vi "Temperature Event Example.vi"() -> ()   [LabVIEW 2012, in "Phidget Temperature Sensor.lvlib"]
uses:
  <instrlib>/Phidgets/Phidget Temperature Sensor/Phidget Temperature Sensor.lvlib
  <instrlib>/Phidgets/Phidget Temperature Sensor/Public/TemperatureSensorStart.vi
  <instrlib>/Phidgets/Phidget Temperature Sensor/Public/TemperatureSensorClose.vi
  <instrlib>/Phidgets/Phidget Common/Phidget Common.lvlib
panel:
  out "Temperature":dbl
  in  "stop":bool
  out "Serial Number Return":i32
  in  "Device Info":T1={"Serial Number"=-1, "Channel"=0, "Port"=0}
  out "error out":errorcluster
  # "Be sure to use this stop button to stop the program.\nIf you use the \"Abort Execution\" button, you will\nneed to use PhidgetResetLibrary.vi or restart Labview \nin order for any Phidgets to work."
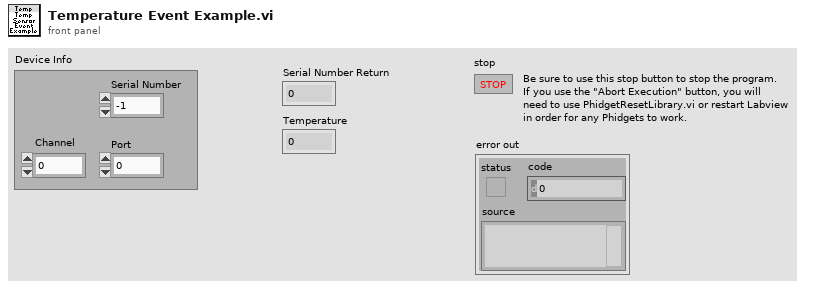
[diagram p1: front panel]
types:
  T1 = cluster{"Serial Number":i32, "Channel":i32, "Port":i32}
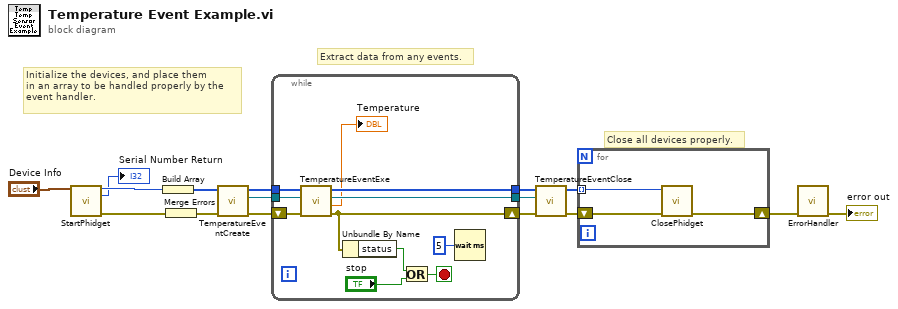
[diagram p0: block diagram]
diagram:
  # "Close all devices properly."
  # "Extract data from any events."
  # "Initialize the devices, and place them\nin an array to be handled properly by the\nevent handler."
  n1 = call-poly <instrlib>:"StartPhidget.vi"("Device Info"="Device Info") -> ("Phidget ID"=w6:u64, "Serial Number Return"=→"Serial Number Return":i32, "error out"=w2:errorcluster)  [unwired: 11 in, 1 out]
  n2 = Build Array(w6) -> (w16:u64[])
  n3 = Merge Errors(w2) -> (w8:errorcluster)
  n4 = call <instrlib>:"TemperatureEventCreate.vi"("error in (no error)"=w8, "Devices In"=w16) -> ("error out"=w10:errorcluster, "Event Registration Refnum"=w3:refnum<event-registration>, "Devices Out"=w15:u64[])  [unwired: 7 in]
  n5 = while {
    tunnel: w15 -> [w27]
    tunnel: [w26] -> w12
    shift-right: [w22] -> w11
    shift-left: w10 -> [w25]
    tunnel: [w23] -> w4
    tunnel: w3 -> [w18]
    stop <- w21 stop-if-true
    n6 = call <instrlib>:"TemperatureEventExe.vi"("error in (no error)"=w25, "Event Registration Refnum In"=w18, "Devices In"=w27) -> ("error out"=w22:errorcluster, "Temperature"=→"Temperature":dbl, "Event Registration Refnum Out"=w26:refnum<event-registration>, "Devices Out"=w23:u64[])  [unwired: 3 in, 2 out]
    n7 = Unbundle By Name(w22) -> ("status"=w19:bool)
    n8 = Or(x=w19, y="stop") -> (x .or. y?=w21:bool)
    n9 = Wait (ms)(milliseconds to wait=u32 5) -> ()  [unwired: 1 out]
  }
  n10 = call <instrlib>:"TemperatureEventClose.vi"("error in (no error)"=w11, "Event Registration Refnum In"=w12, "Devices In"=w4) -> ("error out"=w7:errorcluster, "Devices Out"=w5:u64[])  [unwired: 7 in]
  n11 = for {
    tunnel: w5 -> [w28] mode=indexing
    shift-right: [w30] -> w14
    shift-left: w7 -> [w29]
    n12 = call-poly <instrlib>:"ClosePhidget.vi"("error in"=w29, "Device In"=w28) -> ("error out"=w30:errorcluster)  [unwired: 9 in]
  }
  n13 = call <instrlib>:"ErrorHandler.vi"("error in"=w14) -> ("error out"=→"error out":errorcluster)  [unwired: 9 in, 1 out]
